vi "Get SS2 HDF5 File Version.vi"(8 "error in (no error)":errorcluster, 11 "path in":path) -> (0 "error out":errorcluster, 2 "File Version":string, 3 "ref out":i32)   [LabVIEW 2021, in "SwissSPAD.lvlib"]
uses:
  <vilib>/addons/h5labview2/base/lib_path.vi
  <vilib>/addons/h5labview2/base/H5Equery.vi
  <vilib>/addons/h5labview2/base/hid_t.ctl
  <vilib>/addons/h5labview2/dataset/H5Dread.llb/H5Dread.xnode
  SwissSPAD.lvlib
  <vilib>/addons/h5labview2/file/H5F.lvlib
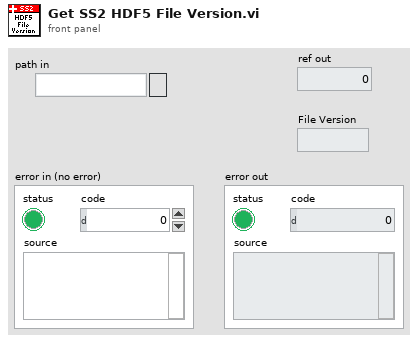
[diagram p1: front panel]
types:
  T1 = typedef "hid_t.ctl" = i64
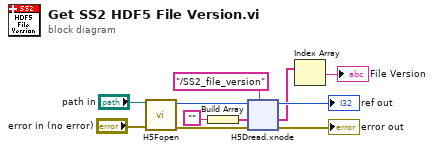
[diagram p0: block diagram]
diagram:
  n1 = call <vilib>:"H5Fopen.vi"("error in (no error)"="error in (no error)", "path"="path in") -> ("error out"=w3:errorcluster, "ref out"=w4:T1)  [unwired: 8 in]
  n2 = Build Array("") -> (w7:string[])
  n3 = xnode "H5Dread.xnode"("dataset name (this)"="/SS2_file_version", "error in (no error)"=w3, "default"=w7, "ref in"=w4) -> ("error out"=→"error out":errorcluster, "data"=w6:string[], "ref out"=→"ref out":T1)  [unwired: 2 in, 1 out]
  n4 = Index Array(array=w6) -> (element=→"File Version":string)  [unwired: 1 in]
